vi "Do.vi"(8 "error in":errorcluster, 10 "Actor in":refnum<class "Actor.lvclass">, 11 "PowerSupply MSG":refnum<class "PowerSupply MSG.lvclass">) -> (0 "error out":errorcluster, 2 "Actor out":refnum<class "Actor.lvclass">)   [LabVIEW 2014, in "Controller.lvlib" / "PowerSupply MSG.lvclass"]
doc: "(<B>Filename</B>: Actor Framework.lvlib:Message.lvclass:Do.vi)\n\nDefines what a message does when it is received by an actor. Generally, a message instructs an actor to invoke one of its methods. By default, this method does nothing. A child class must override it to define behavior. Create a child class by using the Actor Framework Message Maker dialog box."
uses:
  PowerSupply MSG.lvclass
  <vilib>/ActorFramework/Actor/Actor.lvclass
  PowerSupply MSG.lvclass/PowerSupply MSG.ctl
  Controller.lvclass
  Controller.lvclass/Controller.ctl
  <vilib>/DAQmx/write.llb/DAQmx Write (Digital 1D Bool NChan 1Samp 1Line).vi
  Accessors/Read log.vi
  <vilib>/DAQmx/miscellaneous.llb/DAQmx Fill In Error Info.vi
  <userlib>/_Session Fwk/Session - Root.lvclass
  reusable/Session APIs/Session Log/System Log.lvclass
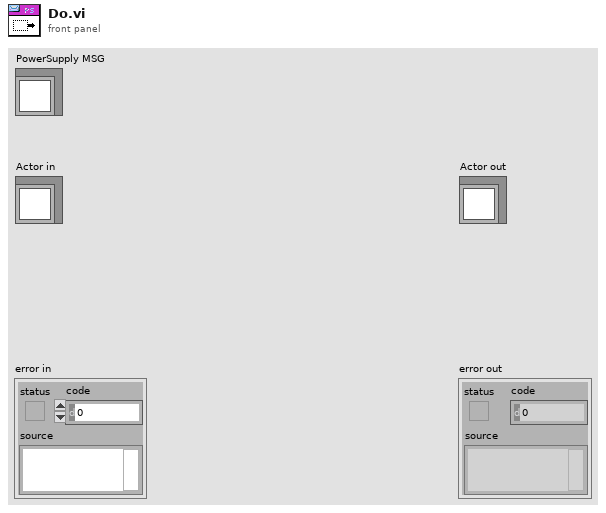
[diagram p1: front panel]
types:
  T1 = typedef "Session - Root.lvclass/Session Handle.ctl" = refnum<data-value>
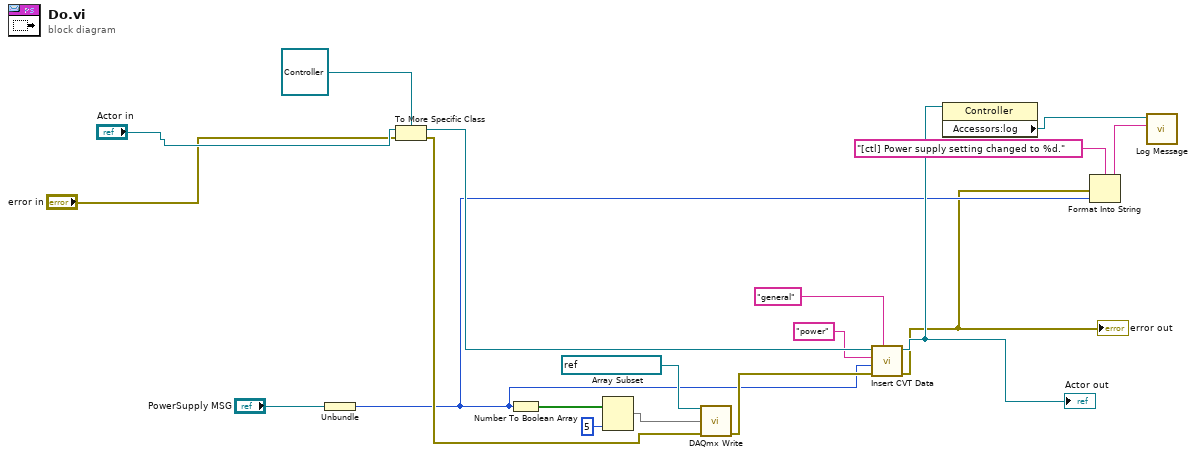
[diagram p0: block diagram]
diagram:
  n1 = Unbundle("PowerSupply MSG") -> (w3:u8)
  n2 = To More Specific Class(target class=refnum<class "Controller.lvclass"> refnum ("Controller.lvlib:Controller"), reference="Actor in", error in="error in") -> (specific class reference=w10:refnum<class "Controller.lvclass">, error out=w7:errorcluster)
  n3 = Number To Boolean Array(number=w3) -> (Boolean array=w19:bool[])
  n4 = Array Subset(array=w19, length=5) -> (w17:bool[])  [unwired: 1 in]
  n5 = call-poly <vilib>:"DAQmx Write.vi"("task/channels in"=refnum<k21> "Power Supply", "data"=w17, "error in"=w7) -> ("error out"=w11:errorcluster)  [unwired: 10 in, 2 out]
  n6 = call "Insert CVT Data.vi"("Group"="general", "error in"=w11, "Data"=w3, "tag"="power", "Controller in"=w10) -> ("error out"=w2:errorcluster, "Controller out"=w6:refnum<class "Controller.lvclass">)  [unwired: 5 in]
  "error out" <- w2
  "Actor out" <- w6
  n7 = property class="Controller"(reference=w6) -> ("Accessors:log"=w5:T1)  [unwired: 1 in, 2 out]
  n8 = Format Into String(format string="[ctl] Power supply setting changed to %d.", error in=w2, w3) -> (resulting string=w1:string)  [unwired: 1 in, 1 out]
  n9 = call "Log Message.vi"("MSG In"=w1, "session in"=w5) -> ()  [unwired: 8 in, 2 out]
